vi "Get DAQ Settings from Config.vi"(8 "error in (no error)":errorcluster, 11 "DAQ":refnum<class "DAQ.lvclass">) -> (0 "error out":errorcluster, 2 "DAQ Settings":T1, 3 "DAQ":refnum<class "DAQ.lvclass">)   [LabVIEW 2022 SP3, in "DAQ.lvclass"]
doc: "Developed by Kevin Thompson\nkevin@thompsonengineering.net\n\nCopyright 2018-2020\nThompson Engineering, LLC"
uses:
  DAQ.lvclass
  DAQ.lvclass/DAQ.ctl
  DataTypes/TD AI InstSettings--cluster.ctl
  Process/ProcessSupport/TD SimAI Ranges--cluster.ctl
  DataTypes/TD DAQ Settings--cluster.ctl
  DataTypes/TD AI Instrument Settings--cluster.ctl
  DataTypes/TD DI Instrument Settings--cluster.ctl
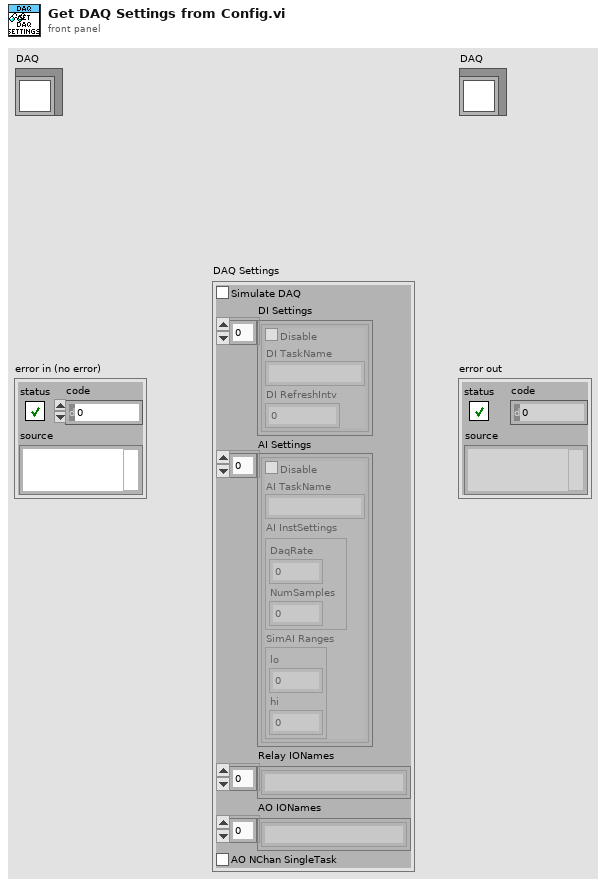
[diagram p1: front panel]
types:
  T1 = typedef "DAQ.lvclass/TD DAQ Settings--cluster.ctl" = cluster{"Simulate DAQ":bool, "DI Settings":T2[], "AI Settings":T3[], "Relay IONames":string[], "AO IONames":string[], "AO NChan SingleTask":bool}
  T2 = typedef "DAQ.lvclass/TD DI Instrument Settings--cluster.ctl" = cluster{"Disable":bool, "DI TaskName":string, "DI RefreshIntv":i32}
  T3 = typedef "DAQ.lvclass/TD AI Instrument Settings--cluster.ctl" = cluster{"Disable":bool, "AI TaskName":string, "AI InstSettings":T4, "SimAI Ranges":T5}
  T4 = typedef "DAQ.lvclass/TD AI InstSettings--cluster.ctl" = cluster{"DaqRate":dbl, "NumSamples":i32}
  T5 = typedef "DAQ.lvclass/TD SimAI Ranges--cluster.ctl" = cluster{"lo":dbl, "hi":dbl}
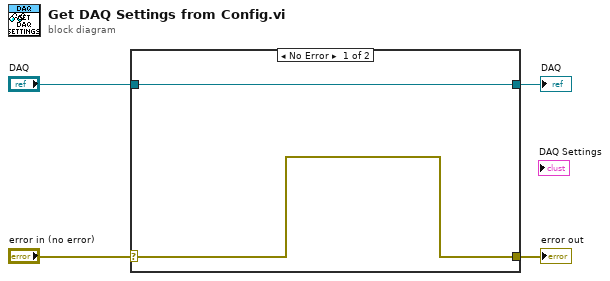
[diagram p0: block diagram]
diagram:
  n1 = case shown="No Error" "error in (no error)" {
    selector: "error in (no error)" -> [w5 w7]
    tunnel: [w5 w7] -> w3
    tunnel: [w6 w8] -> w1
    tunnel: "DAQ" -> [w6 w8]
    frame No Error {
    }
    frame Error {
    }
  }
  "error out" <- w3
  "DAQ" <- w1
